vi "Tank Drive.vi"() -> ()   [LabVIEW 2013]
doc: "Tank Drive Example\n\nThis example shows how to implement tank drive and uses two joysticks for input."
uses:
  <vilib>/Rock Robotics/WPI/Joystick/WPI_JoystickDeviceEnum.ctl
  <vilib>/Rock Robotics/SystemInterfaces/DIO/FPGA_DIOChannel.ctl
  <vilib>/Rock Robotics/SystemInterfaces/Typedef/FPGA_TypedefDigitalModule.ctl
  <vilib>/Rock Robotics/SystemInterfaces/DIO/FPGA_DIORelayChannel.ctl
  <vilib>/Rock Robotics/SystemInterfaces/DIO/FPGA_DIOPWMChannel.ctl
  Robot_Framework_2014/SingleSolenoidAction.ctl
  <vilib>/Rock Robotics/SystemInterfaces/Typedef/FPGA_TypedefSolenoidModule.ctl
  <vilib>/Rock Robotics/WPI/Solenoid/WPI_SolenoidChannel.ctl
  <vilib>/Rock Robotics/WPI/RobotDrive/WPI_RobotDriveOpen2MotorWithTalon.vi
  <vilib>/Rock Robotics/WPI/Solenoid/WPI_SolenoidOpenSingle.vi
panel:
  in  "stop":bool
  # "Set these inputs before running."
  # "Wiring Diagram for Digital Sidecar connected to an NI 9403 in slot 4"
  # "Digital Sidecar"
  # "Power\nTerminals"
  # "Motor\nTerminals"
  # "PWM cable"
  # "This shows wiring for a Luminary Micro Jaguar speed controller.  The wiring is similar for a Victor speed controller.  For a Victor, you must also select the appropriate instance of the Motor Open VI on the diagram.  This is only the wiring for the Left Motor.  The Right Motor would be similarly wired to PWM Channel 2."
  # "PWR"
  # "SIG"
  # "(-)"
  # "+V"
  # "10"
  # "9"
  # "8"
  # "7"
  # "6"
  # "5"
  # "4"
  # "3"
  # "2"
  # "1"
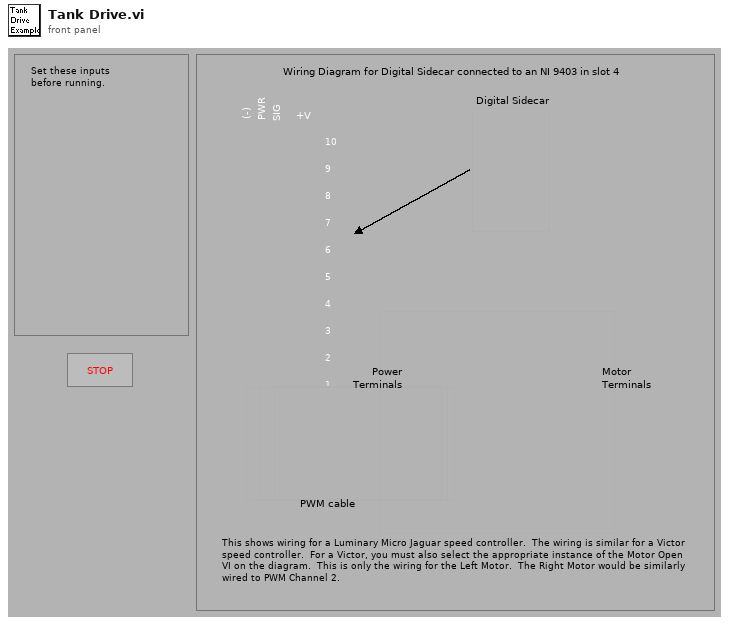
[diagram p1: front panel]
types:
  T1 = typedef "WPI_SolenoidChannel.ctl" = enum8{"Solenoid 1", "Solenoid 2", "Solenoid 3", "Solenoid 4", "Solenoid 5", "Solenoid 6", "Solenoid 7", "Solenoid 8", "Invalid"}
  T2 = typedef "FPGA_TypedefSolenoidModule.ctl" = enum16{"Solenoid Module 1", "Solenoid Module 2"}
  T3 = typedef "SingleSolenoidAction.ctl" = enum16{"Init", "SetState", "Disable"}
  T4 = typedef "FPGA_DIOPWMChannel.ctl" = enum8{"PWM 1", "PWM 2", "PWM 3", "PWM 4", "PWM 5", "PWM 6", "PWM 7", "PWM 8", "PWM 9", "PWM 10", "Invalid"}
  T5 = typedef "FPGA_DIORelayChannel.ctl" = enum8{"Relay 1", "Relay 2", "Relay 3", "Relay 4", "Relay 5", "Relay 6", "Relay 7", "Relay 8", "Invalid"}
  T6 = typedef "FPGA_TypedefDigitalModule.ctl" = enum16{"Digital Module 1", "Digital Module 2"}
  T7 = typedef "FPGA_DIOChannel.ctl" = enum8{"DIO 1", "DIO 2", "DIO 3", "DIO 4", "DIO 5", "DIO 6", "DIO 7", "DIO 8", "DIO 9", "DIO 10", "DIO 11", "DIO 12", "DIO 13", "DIO 14", "Invalid"}
  T8 = typedef "WPI_JoystickDeviceEnum.ctl" = enum16{"USB 1", "USB 2", "USB 3", "USB 4", "Kinect 1", "Kinect 2"}
  T9 = typedef "WPI_SolenoidDevRef.ctl" = cluster{"DevStatus":errorcluster, "Solenoid Module":T2, "Forward Solenoid Channel":T1, "Reverse Solenoid Channel":T1}
  T10 = typedef "WPI_JoystickDevRef.ctl" = cluster{"Device":T8}
  T11 = typedef "WPI_RobotDriveDevRef.ctl" = cluster{"DevStatus":errorcluster, "Motors[]":T12[], "Square Inputs":bool, "Max Output":dbl, "Isochronous":bool}
  T12 = typedef "WPI_MotorControlDeviceRef.ctl" = cluster{"DeviceStatus":errorcluster, "Type":enum16{"PWM", "CAN"}, "PWM":cluster{"Digital Module":T6, "PWM Channel":T4, "DeadBand":T13}, "CAN":cluster{"Device Number":u8, "Control Mode":T14, "Semaphore":T15, "Max Vout":dbl}, "Invert":bool, "TransformRef":T16, "InvTransformRef":T16}
  T13 = typedef "WPI_PWMDeadband.ctl" = cluster{"Name":string, "maxPositivePwm":i32, "minPositivePwm":i32, "centerPwm":i32, "maxNegativePwm":i32, "minNegativePwm":i32, "angularRange":u16}
  T14 = typedef "WPI_CANJaguar_ControlMode.ctl" = enum8{"Percent VBus", "Current", "Speed", "Position", "Voltage"}
  T15 = typedef "Semaphore RefNum" = refnum<k1>
  T16 = typedef "WPI_PWMTransform_ConPane.ctl" = refnum<vi>
  T17 = typedef "WPI_JoystickButtonState.ctl" = cluster{"Button 1":bool, "Button 2":bool, "Button 3":bool, "Button 4":bool, "Button 5":bool, "Button 6":bool, "Button 7":bool, "Button 8":bool, "Button 9":bool, "Button 10":bool, "Button 11":bool, "Button 12":bool}
  T18 = cluster{"axis 1 (x)":dbl, "axis 2 (y)":dbl, "axis 3 (throttle)":dbl, "axis 4":dbl, "axis 5":dbl, "axis 6":dbl}
  T19 = typedef "WPI_CompressorDevRef.ctl" = cluster{"DevStatus":errorcluster, "DigitalInputDevRef":T20, "RelayDevRef":T21}
  T20 = typedef "WPI_DigitalInputDevRef.ctl" = cluster{"DevStatus":errorcluster, "DIO Channel":T7, "Digital Module":T6}
  T21 = typedef "WPI_RelayDevRef.ctl" = cluster{"DevStatus":errorcluster, "Relay Channel":T5, "Digital Module":T6, "Relay Direction":T22}
  T22 = typedef "WPI_RelayDirection.ctl" = enum16{"Both directions", "Forward only", "Reverse only"}
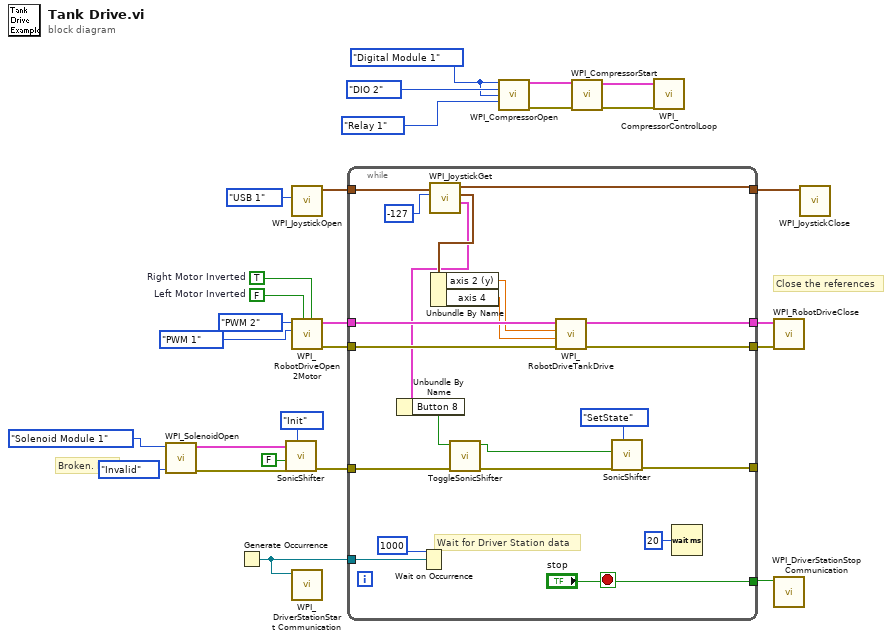
[diagram p0: block diagram]
diagram:
  w17 = FPGA_TypedefDigitalModule."Digital Module 1" ("Pressure Switch Digital Module (Module 1)")
  w22 = TRUE  # Right Motor Inverted
  w23 = FALSE  # Left Motor Inverted
  # "Broken. Fix."
  # "Close the references"
  n1 = call-poly <vilib>:"WPI_SolenoidOpen.vi"("Solenoid Channel"=WPI_SolenoidChannel."Invalid", "Solenoid Module (Module 1)"=FPGA_TypedefSolenoidModule."Solenoid Module 1") -> ("error out"=w5:errorcluster, "SolenoidDevRef"=w3:T9)  [unwired: 8 in]
  n2 = Generate Occurrence() -> (w25:refnum<k4>)
  n3 = call "SonicShifter.vi"("Action"=SingleSolenoidAction."Init", "error in (no error)"=w5, "Default Position"=FALSE, "SolenoidDevRef"=w3) -> ("error out"=w7:errorcluster)  [unwired: 7 in]
  n4 = call <vilib>:"WPI_JoystickOpen.vi"("JoystickDevice"=WPI_JoystickDeviceEnum."USB 1") -> ("JoystickDevRef"=w21:T10)  [unwired: 10 out]
  n5 = call-poly <vilib>:"WPI_RobotDriveOpen2Motor.vi"("Right Motor Inverted"=w22, "Left Motor Inverted"=w23, "Right Motor"=FPGA_DIOPWMChannel."PWM 1", "Left Motor"=FPGA_DIOPWMChannel."PWM 2") -> ("error out"=w9:errorcluster, "RobotDriveDevRef"=w27:T11)  [unwired: 1 in, 5 out]
  n6 = call <vilib>:"WPI_DriverStationStart Communication.vi"("occurrence"=w25) -> ()  [unwired: 11 out]
  n7 = while {
    tunnel: w27 -> [w44]
    tunnel: [w45] -> w26
    tunnel: w25 -> [w48]
    tunnel: ["stop"] -> w24
    tunnel: w21 -> [w43]
    tunnel: [w38] -> w19
    tunnel: w9 -> [w37]
    tunnel: [w36] -> w8
    tunnel: [w32] -> _
    tunnel: w7 -> [w31]
    stop <- "stop" stop-if-true
    # "Wait for Driver Station data"
    n8 = Wait on Occurrence(2:w48, 3:1000 ("ms timeout (-1)")) -> ()  [unwired: 2 out]
    n9 = call <vilib>:"WPI_JoystickGet.vi"("Scaler"=i8 -127, "JoystickDevRef"=w43) -> ("Buttons"=w30:T17, "Axes"=w39:T18, "JoystickDevRef"=w38:T10)  [unwired: 3 in]
    n10 = Unbundle By Name(w30) -> ("Button 8"=w29:bool)
    n11 = Unbundle By Name(w39) -> ("axis 2 (y)"=w41:dbl, "axis 4"=w40:dbl)
    n12 = call "ToggleSonicShifter.vi"("error in"=w31, "cSonicShifter"=w29) -> ("error out"=w34:errorcluster, "Actuate?"=w35:bool)  [unwired: 8 in]
    n13 = call <vilib>:"WPI_RobotDriveTankDrive.vi"("error in (no error)"=w37, "Right axis value"=w40, "Left axis value"=w41, "RobotDriveDevRef"=w44) -> ("error out"=w36:errorcluster, "RobotDriveDevRef"=w45:T11)  [unwired: 6 out]
    n14 = call "SonicShifter.vi"("Action"=SingleSolenoidAction."SetState", "error in (no error)"=w34, "Actuate?"=w35) -> ("error out"=w32:errorcluster)  [unwired: 8 in]
    n15 = Wait (ms)(milliseconds to wait=u32 20) -> ()  [unwired: 1 out]
  }
  n16 = call <vilib>:"WPI_CompressorOpen.vi"("Pressure Switch Digital Module (Module 1)"=w17, "Pressure Switch DIO Channel"=FPGA_DIOChannel."DIO 2", "Relay Digital Module (Module 1)"=w17, "Relay Channel"=FPGA_DIORelayChannel."Relay 1") -> ("CompressorDevRef"=w15:T19, "error out"=w13:errorcluster)  [unwired: 10 in]
  n17 = call <vilib>:"WPI_CompressorStart.vi"("error in (no error)"=w13, "CompressorDevRef"=w15) -> ("error out"=w12:errorcluster, "CompressorDevRef"=w14:T19)  [unwired: 8 in]
  n18 = call <vilib>:"WPI_CompressorControlLoop.vi"("error in (no error)"=w12, "CompressorDevRef"=w14) -> ()  [unwired: 10 in]
  n19 = call <vilib>:"WPI_RobotDriveClose.vi"("error in (no error)"=w8, "RobotDriveDevRef"=w26) -> ()  [unwired: 10 out]
  n20 = call <vilib>:"WPI_DriverStationStop Communication.vi"("StopCommunication"=w24) -> ()  [unwired: 1 in, 10 out]
  n21 = call <vilib>:"WPI_JoystickClose.vi"("JoystickDevRef"=w19) -> ()  [unwired: 11 out]
